vi "Enqueue File.vi"(10 "filepath":path, 11 "Blocks queue":refnum<queue>) -> (2 "error out":errorcluster)   [LabVIEW 2013, in "SHA-1.lvlib" / "SHA-1.lvclass"]
uses:
  SHA-1.lvclass
  Data-vector.ctl
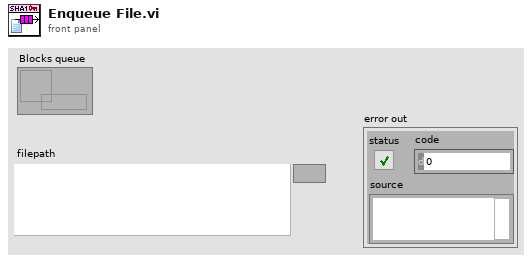
[diagram p1: front panel]
types:
  T1 = enum16{"open", "replace", "create", "open or create", "replace or create", "replace or create with confirmation"}
  T2 = typedef "SHA-1.lvlib/SHA-1.lvclass/Data-vector.ctl" = cluster{"Data[ ]":u8[], "end":bool}
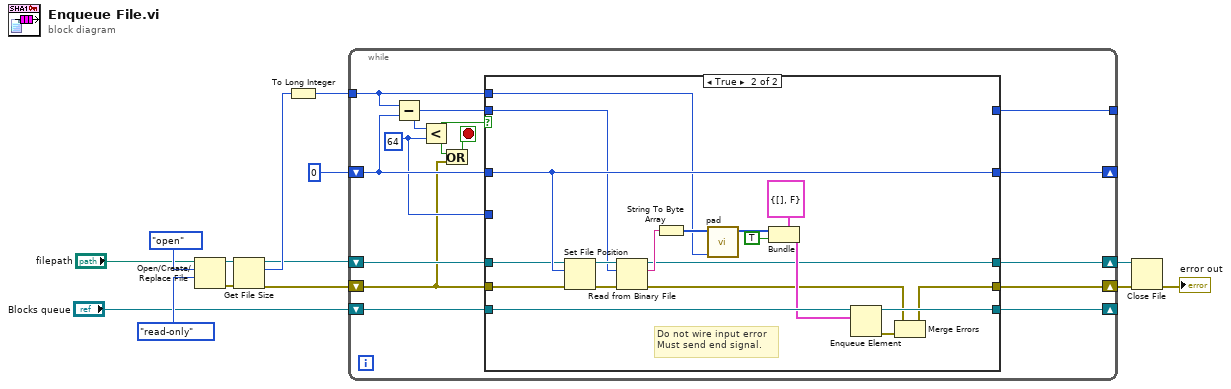
[diagram p0: block diagram]
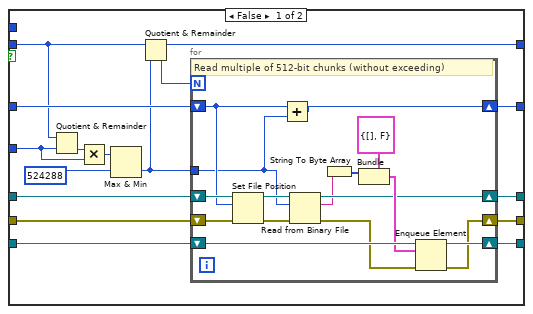
[diagram p2: hidden frame]
diagram:
  n1 = Open/Create/Replace File(file path (use dialog)="filepath", operation (0:open)=T1."open", access (0:read/write)=enum16{"read/write", "read-only", "write-only"}."read-only") -> (refnum out=w13:refnum<file>, error out=w12:errorcluster)  [unwired: 3 in, 1 out]
  n2 = Get File Size(file=w13, error in=w12) -> (refnum out=w7:refnum<file>, size (in bytes)=w9:i64, 0:w6:errorcluster)
  n3 = To Long Integer(number=w9) -> (32bit integer=w8:i32)
  n4 = while {
    shift-right: [w24] -> _
    shift-left: 0 ("offset") -> [w26]
    tunnel: w8 -> [w20]
    tunnel: [w25] -> _
    shift-right: [w27] -> _
    shift-left: "Blocks queue" -> [w28]
    shift-right: [w19] -> w5
    shift-left: w7 -> [w23]
    shift-right: [w18] -> w4
    shift-left: w6 -> [w17]
    stop <- w15 stop-if-true
    w21 = 64 ("y")
    n5 = Subtract(x=w20, y=w26) -> (x-y=w22:i32)
    n6 = Less?(x=w22, y=w21) -> (x < y?=w16:bool)
    n7 = Or(x=w16, y=w17) -> (x .or. y?=w15:bool)
    n8 = case shown="True" w16 {
      tunnel: w28 -> [w44 w79]
      tunnel: [w43 w78] -> w27
      tunnel: w26 -> [w42 w75]
      tunnel: [w36 _] -> w25
      tunnel: [w35 w75] -> w24
      tunnel: w23 -> [w34 w74]
      tunnel: w22 -> [w33 w70]
      tunnel: w21 -> [w32 _]
      tunnel: w20 -> [_ w61]
      tunnel: [w31 w69] -> w19
      tunnel: w17 -> [w30 w68]
      tunnel: [w29 w65] -> w18
      frame False {
        n9 = Quotient & Remainder(x=w33, y=w32) -> (floor(x/y)=w41:i32)  [unwired: 1 out]
        n10 = Multiply(x=w41, y=w32) -> (x*y=w40:i32)
        n11 = Max & Min(x=w40, y=524288) -> (min(x,y)=w37:i32)  [unwired: 1 out]
        n12 = Quotient & Remainder(x=w33, y=w37) -> (x-y*floor(x/y)=w36:i32, floor(x/y)=w38:i32)
        n13 = for {
          N: w38 -> [_]
          shift-right: [w59] -> w43
          shift-left: w44 -> [w60]
          shift-right: [w57] -> w35
          shift-left: w42 -> [w54]
          tunnel: w37 -> [w52]
          shift-right: [w51] -> w31
          shift-left: w34 -> [w56]
          shift-right: [w46] -> w29
          shift-left: w30 -> [w49]
          # "Read multiple of 512-bit chunks (without exceeding)"
          n14 = Set File Position(offset (in bytes) (0)=w54, refnum=w56, error in=w49) -> (refnum out=w53:refnum<file>, error out=w48:errorcluster)  [unwired: 1 in]
          n15 = Add(x=w54, y=w52) -> (x+y=w57:i32)
          n16 = Read from Binary File(8:w48, 10:w52, 11:w53) -> (0:w47:errorcluster, 2:w50:string, 3:w51:refnum<file>)  [unwired: 3 in, 1 out]
          n17 = String To Byte Array(string=w50) -> (unsigned byte array=w55:u8[])
          n18 = Bundle(cluster=T2 {"Data[ ]"=[], "end"=FALSE}, "Data[ ]"=w55) -> (w58:T2)  [unwired: 1 in]
          n19 = Enqueue Element(queue=w60, element=w58, error in (no error)=w47) -> (queue out=w59:refnum<queue>, error out=w46:errorcluster)  [unwired: 1 in, 1 out]
        }
      }
      frame True {
        # "Do not wire input error\nMust send end signal."
        n20 = Set File Position(offset (in bytes) (0)=w75, refnum=w74, error in=w68) -> (refnum out=w72:refnum<file>, error out=w73:errorcluster)  [unwired: 1 in]
        n21 = Read from Binary File(8:w73, 10:w70, 11:w72) -> (0:w66:errorcluster, 2:w71:string, 3:w69:refnum<file>)  [unwired: 3 in, 1 out]
        n22 = String To Byte Array(string=w71) -> (unsigned byte array=w63:u8[])
        n23 = call "pad.vi"("data length"=w61, "Last Block"=w63) -> ("Padding"=w62:u8[])  [unwired: 8 in, 1 out]
        n24 = Bundle(cluster=T2 {"Data[ ]"=[], "end"=FALSE}, "Data[ ]"=w62, "end"=TRUE) -> (w76:T2)
        n25 = Enqueue Element(queue=w79, element=w76) -> (queue out=w78:refnum<queue>, error out=w67:errorcluster)  [unwired: 2 in, 1 out]
        n26 = Merge Errors(w66, w67) -> (w65:errorcluster)
      }
    }
  }
  n27 = Close File(refnum=w5, error in=w4) -> (error out=→"error out":errorcluster)  [unwired: 1 out]
